vi "Build histogram of peaks.vi"(10 "Peaks":dbl[](array[numeric]), 11 "Hours of peaks":i32[](array[numeric])) -> (1 "nbr of elements":i32[](array[numeric]), 2 "%":dbl[](array[numeric]) format="%#_2g", 3 "Peaks":cluster{i32[], dbl[]}[](graph))   [LabVIEW 2018]
panel:
  out "XY Graph":cluster{"Hours of peaks":i32[], "Peaks":dbl[]}(graph)
  out "Start":i32[](array[numeric])=[28800, 36000, 43200, 50400, 57600, 64800, 72000, 79200] format="%<%H:%M>t"
  out "End hours":i32[](array[numeric])=[28800, 36000, 43200, 50400, 57600, 64800, 72000, 79200] format="%<%H:%M>t"
  out "Waveform Graph 2":dbl[](graph)
  out "hours of the peaks":i32[](graph)
  out "End hours":i32[](array[numeric])
  out "Start":i32[](array[numeric])
  # "These numbers are used just to define the case strucutre\nto make the peak analisys on the hours."
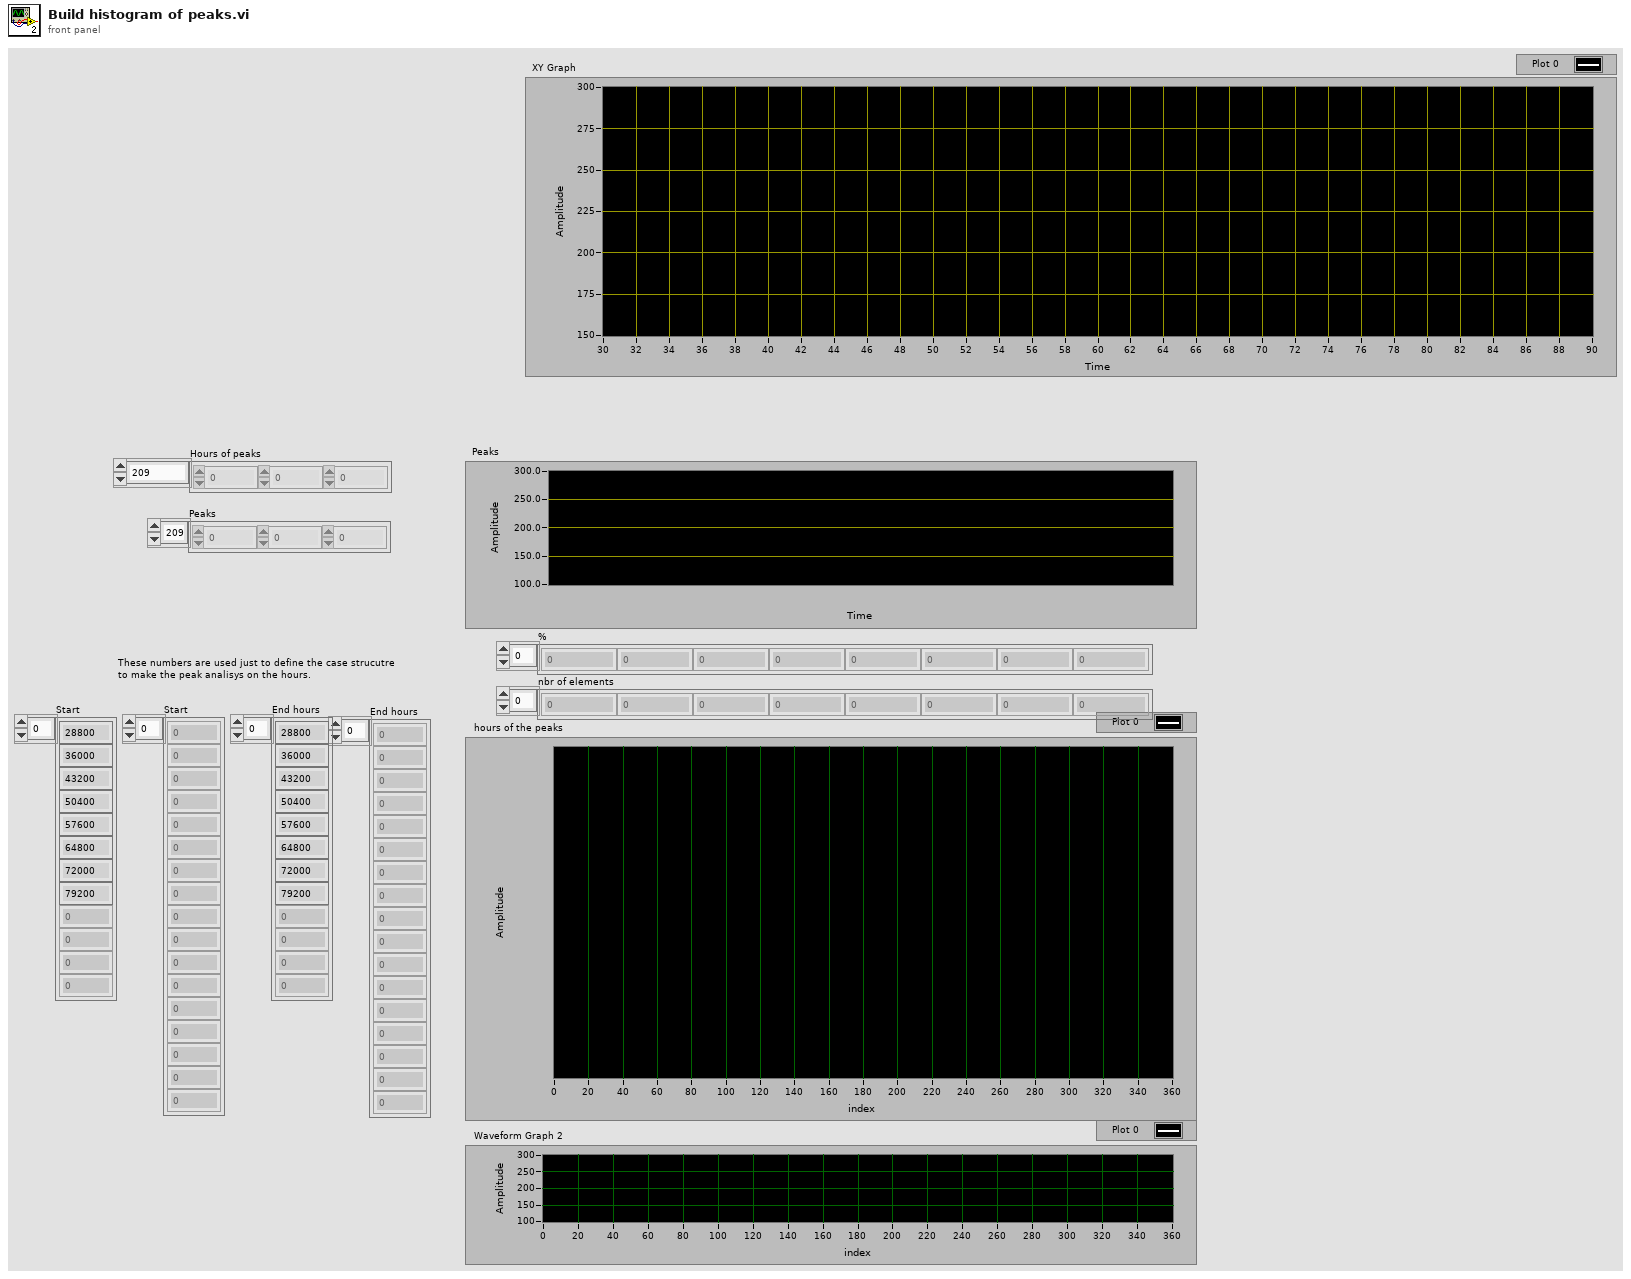
[diagram p1: front panel]
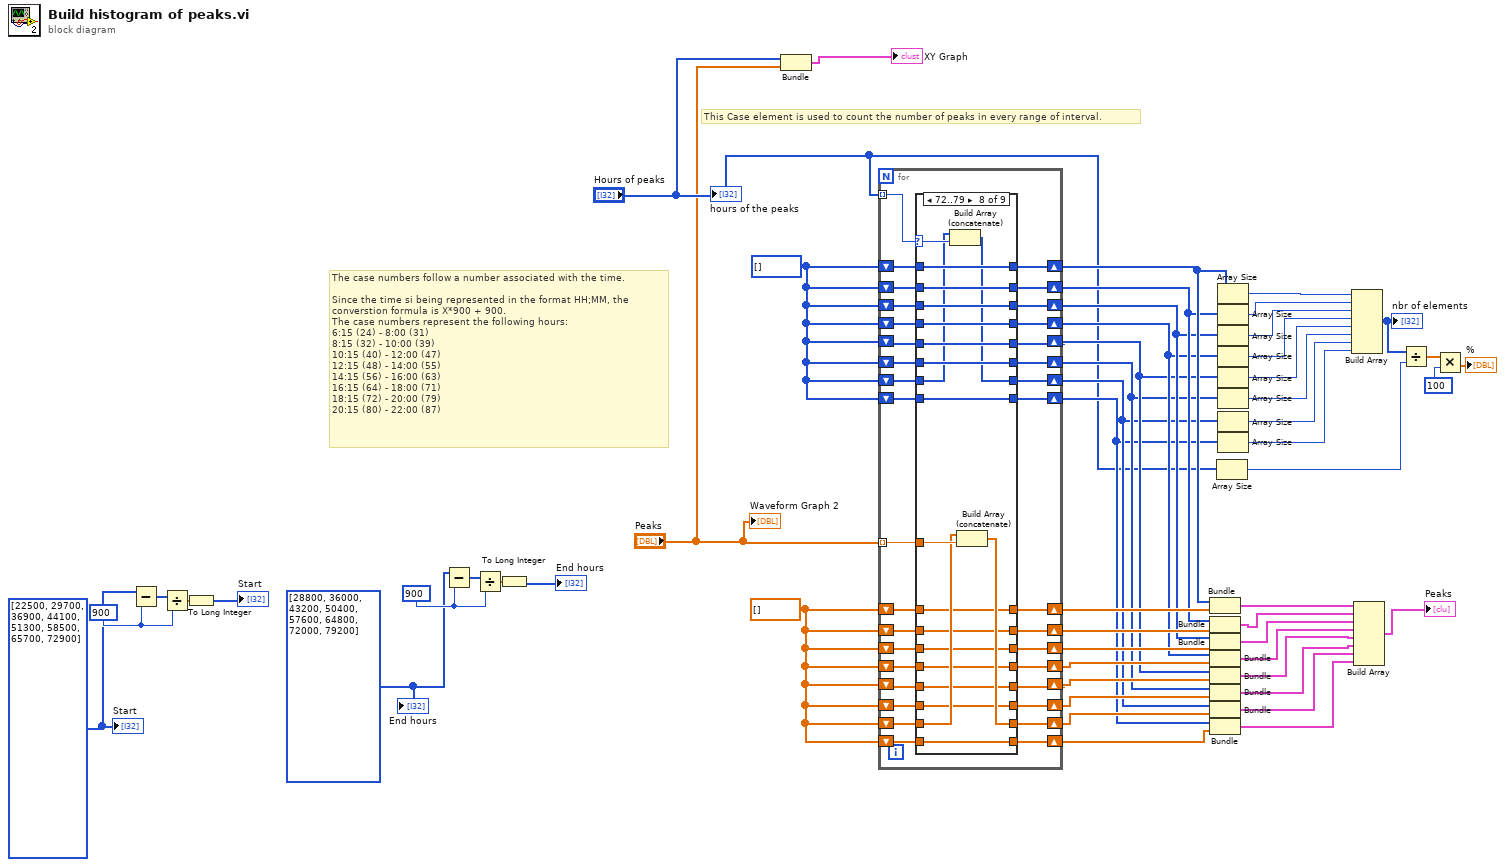
[diagram p0: block diagram]
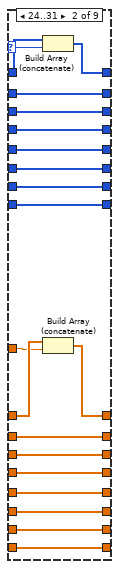
[diagram p3: hidden frame]
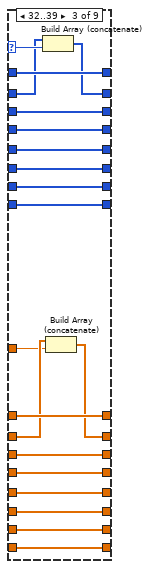
[diagram p4: hidden frame]
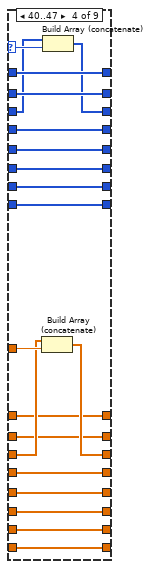
[diagram p5: hidden frame]
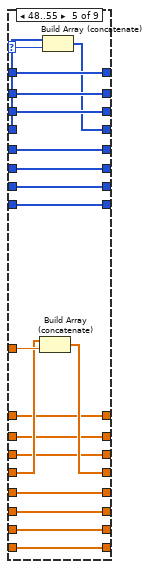
[diagram p6: hidden frame]
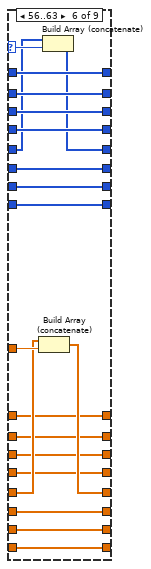
[diagram p7: hidden frame]
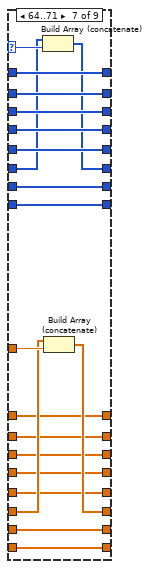
[diagram p8: hidden frame]
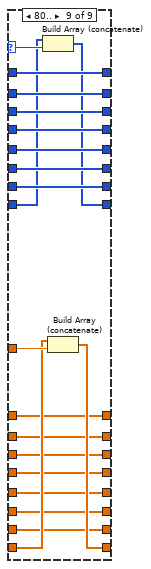
[diagram p9: hidden frame]
diagram:
  w5 = i32[] [22500, 29700, 36900, 44100, 51300, 58500, 65700, 72900] ("Start Hours")
  w47 = i32[] [28800, 36000, 43200, 50400, 57600, 64800, 72000, 79200] ("End hours")
  w31 = dbl[] []
  w44 = i32[] []
  w49 = 900 ("intervals")
  w52 = 900 ("intervals")
  # "The case numbers follow a number associated with the time.\n\nSince the time si being represented in the format HH;MM, the converstion formula is X*900 + 900.\nThe case numbers represent the following hours:\n6:15 (24) - 8:00 (31)\n8:15 (32) - 10:00 (39)\n10:15 (40) - 12:00 (47)\n12:15 (48) - 14:00 (55)\n14:15 (56) - 16:00 (63)\n16:15 (64) - 18:00 (71)\n18:15 (72) - 20:00 (79)\n20:15 (80) - 22:00 (87)"
  # "This Case element is used to count the number of peaks in every range of interval."
  n1 = Subtract(x=w5, y=w52) -> (x-y=w53:i32[])
  n2 = Divide(x=w53, y=w52) -> (x/y=w51:dbl[])
  n3 = To Long Integer(number=w51) -> (32bit integer=→"Start":i32[])
  n4 = Subtract(x=w47, y=w49) -> (x-y=w48:i32[])
  n5 = Divide(x=w48, y=w49) -> (x/y=w50:dbl[])
  n6 = To Long Integer(number=w50) -> (32bit integer=→"End hours":i32[])
  n7 = Bundle("Hours of peaks"="Hours of peaks", "Peaks"="Peaks") -> (→"XY Graph":cluster{"Hours of peaks":i32[], "Peaks":dbl[]})  [unwired: 1 in]
  n8 = for {
    tunnel: "Hours of peaks" -> [w87] mode=indexing
    shift-right: [w85] -> w29
    shift-left: w44 -> [w86]
    shift-right: [w84] -> w21
    shift-left: w44 -> [w83]
    shift-right: [w82] -> w20
    shift-left: w44 -> [w81]
    shift-right: [w80] -> w19
    shift-left: w44 -> [w79]
    shift-right: [w78] -> w18
    shift-left: w44 -> [w77]
    shift-right: [w76] -> w17
    shift-left: w44 -> [w75]
    shift-right: [w74] -> w16
    shift-left: w44 -> [w73]
    shift-right: [w72] -> w15
    shift-left: w44 -> [w71]
    shift-right: [w56] -> w30
    shift-left: w31 -> [w55]
    shift-right: [w57] -> w28
    shift-left: w31 -> [w58]
    shift-right: [w59] -> w27
    shift-left: w31 -> [w60]
    shift-right: [w61] -> w26
    shift-left: w31 -> [w62]
    shift-right: [w63] -> w25
    shift-left: w31 -> [w64]
    shift-right: [w65] -> w24
    shift-left: w31 -> [w66]
    shift-right: [w67] -> w23
    shift-left: w31 -> [w68]
    shift-right: [w69] -> w22
    shift-left: w31 -> [w70]
    tunnel: "Peaks" -> [w54] mode=indexing
    n9 = case shown="72..79" w87 {
      selector: w87 -> [_ w123 w143 w163 w183 w203 w223 w243 w263]
      tunnel: w86 -> [w103 w122 w136 w157 w177 w197 w217 w237 w257]
      tunnel: [w103 w121 w136 w157 w177 w197 w217 w237 w257] -> w85
      tunnel: [w102 w120 w134 w156 w176 w196 w216 w236 w256] -> w84
      tunnel: w83 -> [w102 w120 w135 w156 w176 w196 w216 w236 w256]
      tunnel: [w101 w119 w142 w154 w182 w202 w222 w242 w262] -> w82
      tunnel: w81 -> [w101 w119 w142 w155 w182 w202 w222 w242 w262]
      tunnel: [w100 w118 w141 w162 w174 w201 w221 w241 w261] -> w80
      tunnel: w79 -> [w100 w118 w141 w162 w175 w201 w221 w241 w261]
      tunnel: [w99 w117 w140 w161 w181 w194 w220 w240 w260] -> w78
      tunnel: w77 -> [w99 w117 w140 w161 w181 w195 w220 w240 w260]
      tunnel: [w98 w116 w139 w160 w180 w200 w214 w239 w259] -> w76
      tunnel: w75 -> [w98 w116 w139 w160 w180 w200 w215 w239 w259]
      tunnel: [w97 w115 w138 w159 w179 w199 w219 w234 w258] -> w74
      tunnel: w73 -> [w97 w115 w138 w159 w179 w199 w219 w235 w258]
      tunnel: [w96 w114 w137 w158 w178 w198 w218 w238 w254] -> w72
      tunnel: w71 -> [w96 w114 w137 w158 w178 w198 w218 w238 w255]
      tunnel: w55 -> [w88 w113 w133 w149 w164 w187 w210 w224 w244]
      tunnel: [w88 w111 w133 w149 w164 w187 w210 w224 w244] -> w56
      tunnel: [w89 w110 w131 w150 w165 w188 w209 w225 w245] -> w57
      tunnel: w58 -> [w89 w110 w132 w150 w165 w188 w209 w225 w245]
      tunnel: [w90 w109 w129 w151 w166 w189 w208 w226 w246] -> w59
      tunnel: w60 -> [w90 w109 w129 w152 w166 w189 w208 w226 w246]
      tunnel: [w91 w108 w128 w148 w171 w190 w207 w227 w247] -> w61
      tunnel: w62 -> [w91 w108 w128 w148 w172 w190 w207 w227 w247]
      tunnel: [w92 w107 w127 w147 w170 w191 w206 w228 w248] -> w63
      tunnel: w64 -> [w92 w107 w127 w147 w170 w192 w206 w228 w248]
      tunnel: [w93 w106 w126 w146 w169 w186 w211 w229 w249] -> w65
      tunnel: w66 -> [w93 w106 w126 w146 w169 w186 w212 w229 w249]
      tunnel: [w94 w105 w125 w145 w168 w185 w205 w231 w250] -> w67
      tunnel: w68 -> [w94 w105 w125 w145 w168 w185 w205 w232 w250]
      tunnel: [w95 w104 w124 w144 w167 w184 w204 w230 w251] -> w69
      tunnel: w70 -> [w95 w104 w124 w144 w167 w184 w204 w230 w252]
      tunnel: w54 -> [_ w112 w130 w153 w173 w193 w213 w233 w253]
      frame -1, Default {
      }
      frame 24..31 {
        n10 = Build Array (concatenate)(w122, w123) -> (w121:i32[])
        n11 = Build Array (concatenate)(w113, w112) -> (w111:dbl[])
      }
      frame 32..39 {
        n12 = Build Array (concatenate)(w135, w143) -> (w134:i32[])
        n13 = Build Array (concatenate)(w132, w130) -> (w131:dbl[])
      }
      frame 40..47 {
        n14 = Build Array (concatenate)(w152, w153) -> (w151:dbl[])
        n15 = Build Array (concatenate)(w155, w163) -> (w154:i32[])
      }
      frame 48..55 {
        n16 = Build Array (concatenate)(w172, w173) -> (w171:dbl[])
        n17 = Build Array (concatenate)(w175, w183) -> (w174:i32[])
      }
      frame 56..63 {
        n18 = Build Array (concatenate)(w192, w193) -> (w191:dbl[])
        n19 = Build Array (concatenate)(w195, w203) -> (w194:i32[])
      }
      frame 64..71 {
        n20 = Build Array (concatenate)(w215, w223) -> (w214:i32[])
        n21 = Build Array (concatenate)(w212, w213) -> (w211:dbl[])
      }
      frame 72..79 {
        n22 = Build Array (concatenate)(w235, w243) -> (w234:i32[])
        n23 = Build Array (concatenate)(w232, w233) -> (w231:dbl[])
      }
      frame 80.. {
        n24 = Build Array (concatenate)(w255, w263) -> (w254:i32[])
        n25 = Build Array (concatenate)(w252, w253) -> (w251:dbl[])
      }
    }
  }
  n26 = Bundle(w29, w30) -> (w14:cluster{i32[], dbl[]})  [unwired: 1 in]
  n27 = Bundle(w21, w28) -> (w13:cluster{i32[], dbl[]})  [unwired: 1 in]
  n28 = Bundle(w20, w27) -> (w12:cluster{i32[], dbl[]})  [unwired: 1 in]
  n29 = Bundle(w19, w26) -> (w11:cluster{i32[], dbl[]})  [unwired: 1 in]
  n30 = Bundle(w18, w25) -> (w10:cluster{i32[], dbl[]})  [unwired: 1 in]
  n31 = Bundle(w17, w24) -> (w9:cluster{i32[], dbl[]})  [unwired: 1 in]
  n32 = Bundle(w16, w23) -> (w8:cluster{i32[], dbl[]})  [unwired: 1 in]
  n33 = Bundle(w15, w22) -> (w7:cluster{i32[], dbl[]})  [unwired: 1 in]
  n34 = Array Size(array="Hours of peaks") -> (size(s)=w35:i32)
  n35 = Array Size(array=w29) -> (size(s)=w43:i32)
  n36 = Array Size(array=w21) -> (size(s)=w42:i32)
  n37 = Array Size(array=w20) -> (size(s)=w41:i32)
  n38 = Array Size(array=w19) -> (size(s)=w40:i32)
  n39 = Array Size(array=w18) -> (size(s)=w39:i32)
  n40 = Array Size(array=w17) -> (size(s)=w38:i32)
  n41 = Array Size(array=w16) -> (size(s)=w37:i32)
  n42 = Array Size(array=w15) -> (size(s)=w36:i32)
  n43 = Build Array(w43, w42, w41, w40, w39, w38, w37, w36) -> (w4:i32[])
  "nbr of elements" <- w4
  n44 = Build Array(w14, w13, w12, w11, w10, w9, w8, w7) -> (→"Peaks":cluster{i32[], dbl[]}[])
  n45 = Divide(x=w4, y=w35) -> (x/y=w34:dbl[])
  n46 = Multiply(x=w34, y=100 ("size(s)")) -> (x*y=→"%":dbl[])
  "hours of the peaks" <- "Hours of peaks"
  "Waveform Graph 2" <- "Peaks"
  "End hours" <- w47
  "Start" <- w5
